vi "TIFF_3_TIFF_Bitmap_Encoder.vi"(8 "error in (no error)":errorcluster, 9 "Cluster":T1) -> (0 "Error Out":errorcluster, 1 "output cluster":T1)   [LabVIEW 2025]
doc: "This software was created to prototype writing metadata to a TIFF file with a single image.\n\n<B>Usage:</B> This software is free to use, copy or plagiariaze. It is provided \"as-is\", and no technical support will be provided. The copyright is retained by NASA Marshall Space Flight Center.\n\n<B>Testing:</B> This software was tested by A) verifying that operations were completed successfully using LabVIEW 2009 on Windows XP, .NET version 4.0 and B) Windows Vista Microsoft Office Picture Manager was able to read and display the output file and C) Windows Vista Windows Photo Gallery was able to read and display the output file and the Description and D) Adobe Photoshop for Macintosh was able to correctly load and display the image and all the metadata.\n\n<B>Note:</B> This software requires .NET version 4.0\n\n<B>Warning:</B> This software will overwrite the destination file if it exists.\n\nThis software originally developed by:\nDerek Mayer\nBAE Systems - Technology Solutions & Services\n308 Voyager Way\nHuntsville, AL 35806\n(256) 890-8000\nwww.mevatec.com\nwww.baesystems.com/TSS\nSeptember 2010"
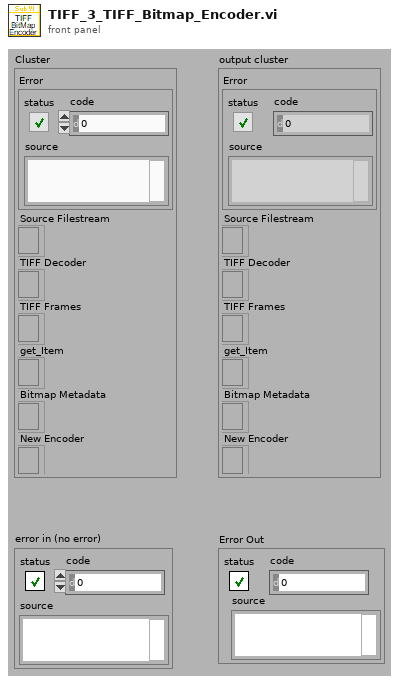
[diagram p1: front panel]
types:
  T1 = cluster{"Error":errorcluster, "Source Filestream":refnum<k24>, "TIFF Decoder":refnum<k24>, "TIFF Frames":refnum<k24>, "get_Item":refnum<k24>, "Bitmap Metadata":refnum<k24>, "New Encoder":refnum<k24>}
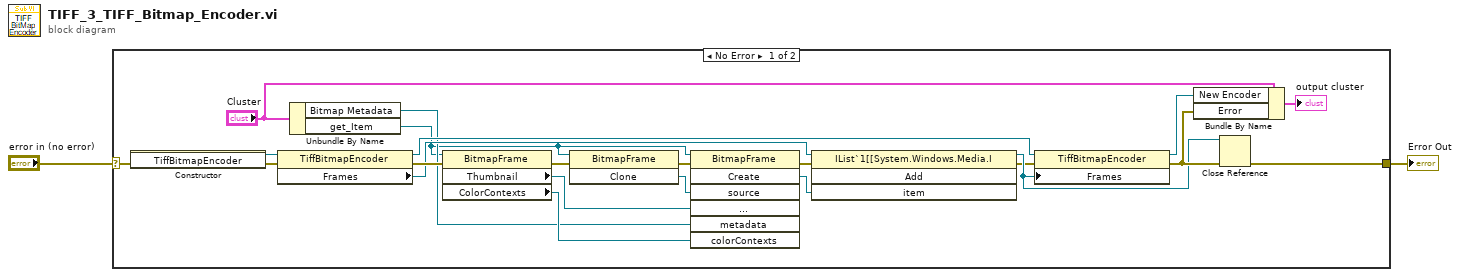
[diagram p0: block diagram]
diagram:
  n1 = case shown="No Error" "error in (no error)" {
    selector: "error in (no error)" -> [w4 w25]
    tunnel: [w3 w25] -> w2
    frame No Error {
      n2 = constructor class="TiffBitmapEncoder"(error in=w4) -> (reference out=w16:refnum<k24>, error out=w24:errorcluster)  [unwired: 2 in, 1 out]
      n3 = property class="TiffBitmapEncoder"(reference=w16, error in=w24) -> (reference out=w20:refnum<k24>, error out=w19:errorcluster, "Frames"=w15:refnum<k24>)
      n4 = Unbundle By Name("Cluster") -> ("Bitmap Metadata"=w11:refnum<k24>, "get_Item"=w9:refnum<k24>)
      n5 = property class="BitmapFrame"(reference=w9, error in=w19) -> (error out=w21:errorcluster, "Thumbnail"=w13:refnum<k24>, "ColorContexts"=w14:refnum<k24>)  [unwired: 1 out]
      n6 = invoke class="BitmapFrame" method="Clone"(reference=w9, error in=w21) -> (error out=w8:errorcluster, "Clone"=w12:refnum<k24>)  [unwired: 1 in, 1 out]
      n7 = invoke class="BitmapFrame" method="Create"(reference=w9, error in=w8, "source"=w12, "thumbnail"=w13, "metadata"=w11, "colorContexts"=w14) -> (error out=w7:errorcluster, "Create"=w10:refnum<k24>)  [unwired: 1 in, 5 out]
      n8 = invoke class="IList`1[[System.Windows.Media.I" method="Add"(reference=w15, error in=w7, "item"=w10) -> (reference out=w18:refnum<k24>, error out=w17:errorcluster)  [unwired: 1 in, 2 out]
      n9 = property class="TiffBitmapEncoder"(reference=w20, error in=w17, "Frames"=w18) -> (reference out=w23:refnum<k24>, error out=w22:errorcluster)
      n10 = Bundle By Name(cluster="Cluster", "New Encoder"=w23, "Error"=w22) -> (→"output cluster":T1)
      n11 = Close Reference(reference=w18, error in (no error)=w22) -> (error out=w3:errorcluster)
    }
    frame Error {
    }
  }
  "Error Out" <- w2
